vi "Get Next.vi"(0 "Subroutine in":refnum<class "Subroutine.lvclass">, 1 "Linked List Ref":refnum<data-value>, 5 "Active Unique ID":string, 9 "Active Element Index":i32, 11 "error in (no error)":errorcluster) -> (3 "Linked List Ref out":refnum<data-value>, 4 "Executioner out":refnum<class "Executioner.lvclass">, 6 "Active Unique ID out":string, 8 "Test Executive Ref out":refnum<data-value>, 10 "Active Element Index out":i32, 12 "Found":bool, 13 "Complete":bool, 14 "Stop":bool, 15 "error out":errorcluster)   [LabVIEW 2017, in "Custom Type Test Executive.lvlib" / "Subroutine.lvclass"]
uses:
  <vilib>/gpm_packages/@cs/test-executive/Source/Custom Type Test Executive/Subroutine/Subroutine.lvclass
  C:/Program Files/National Instruments/LabVIEW 2017/vi.lib/gpm_packages/@cs/test-executive/Source/Test Executive/Executioner/Executioner.lvclass
  <vilib>/gpm_packages/@cs/test-executive/Source/Test Executive/Executioner/Executioner.lvclass
  <vilib>/gpm_packages/@cs/linked-list/Source/Linked List/ILinkedList/ILinked List.lvclass
  <vilib>/gpm_packages/@cs/test-executive/Source/Test Executive/ITestExecutive/ITest Executive.lvclass
  <vilib>/gpm_packages/@cs/test-executive/Source/Custom Type Test Executive/Test Executive Data Type/Test Executive.lvclass/Test Executive.ctl
  <vilib>/gpm_packages/@cs/data-type-serializer/source/String/String.lvclass/String.ctl
  8685ad62-a5f1-424e-9210-060c18869b42.vi
  73af2345-b58a-4bc3-bab0-c6c44c39e3df.vi
  cb17b2c6-08af-4f3d-87c2-f0635200e88a.vi
  b989164a-f16b-4661-a128-dada9db9fdaa.vi
  56bd1768-b4b8-4ab7-8904-4290c8f45432.vi
  0b71244f-90f5-4307-84d1-8667a03d3b22.vi
  <vilib>/gpm_packages/@cs/test-executive/Source/Custom Type Test Executive/Test Executive Data Type/Test Executive.lvclass
  C:/Program Files/National Instruments/LabVIEW 2017/vi.lib/gpm_packages/@cs/data-type-serializer/source/Data Type/Data Type.lvclass
  <vilib>/gpm_packages/@cs/data-type-serializer/source/String/String.lvclass
  <vilib>/Utility/error.llb/Error Cluster From Error Code.vi
  <vilib>/gpm_packages/@cs/linked-list/Source/Linked List/Linked List Ref/Linked List Ref.lvclass
  <vilib>/gpm_packages/@cs/test-executive/Source/Test Executive/TestExecutive Ref/TestExecutive Ref.lvclass
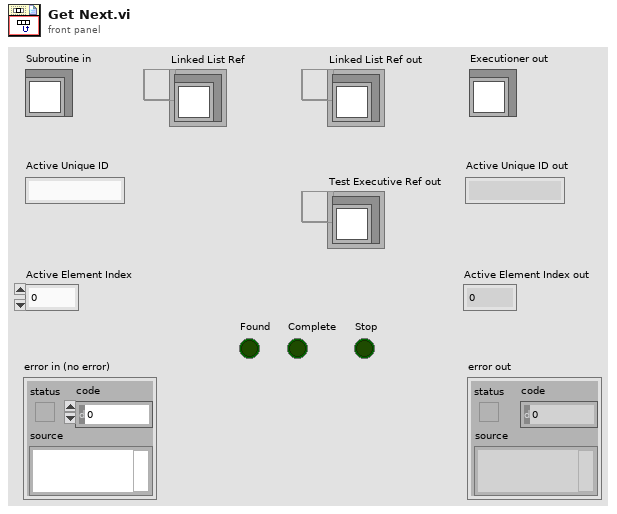
[diagram p1: front panel]
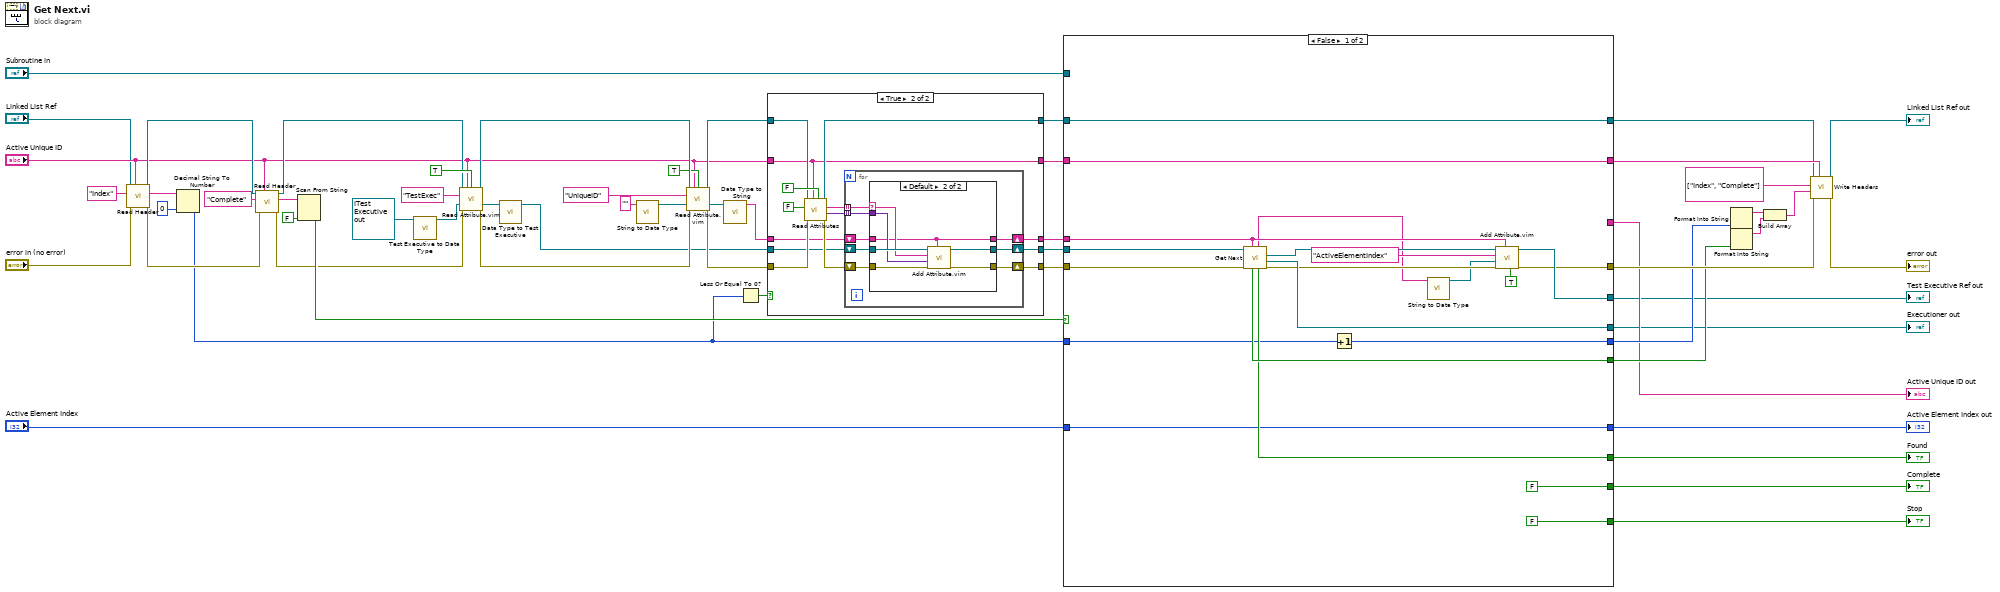
[diagram p0: block diagram]
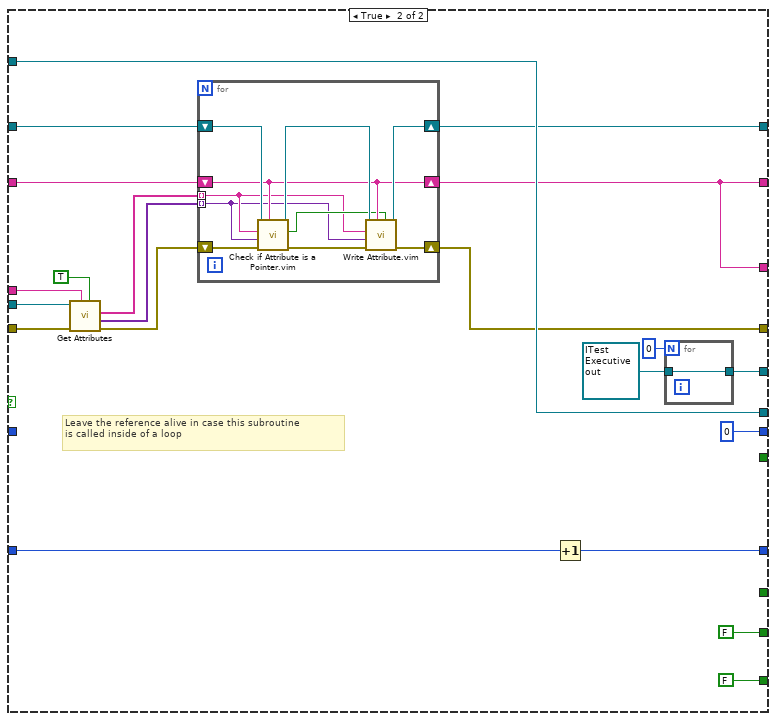
[diagram p4: hidden frame]
diagram:
  n1 = call <vilib>:"Read Header.vi"("Linked List ID"="Active Unique ID", "error in (no error)"="error in (no error)", "Header Name"="Index" ("Attribute Name"), "Linked List Ref"="Linked List Ref") -> ("error out"=w44:errorcluster, "Header Value"=w50:string, "Linked List Ref out"=w45:refnum<data-value>)  [unwired: 4 in, 1 out]
  n2 = Decimal String To Number(string=w50, default (0L)=0 ("Attribute")) -> (number=w23:i32)  [unwired: 1 in, 1 out]
  n3 = call <vilib>:"Read Header.vi"("Linked List ID"="Active Unique ID", "error in (no error)"=w44, "Header Name"="Complete" ("Attribute Name"), "Linked List Ref"=w45) -> ("error out"=w32:errorcluster, "Header Value"=w47:string, "Linked List Ref out"=w33:refnum<data-value>)  [unwired: 4 in, 1 out]
  n4 = Scan From String(input string=w47, default 1=FALSE) -> (output 1=w52:bool)  [unwired: 3 in, 3 out]
  n5 = call <vilib>:"Test Executive to Data Type.vi"("Test Executive Ref"=refnum<data-value> refnum ("Test Executive Ref out")) -> ("Boolean out"=w3:refnum<class "Test Executive.lvclass">)  [unwired: 9 in, 1 out]
  n6 = call "Read Attribute.vim"("Linked List Ref"=w33, "Linked List ID"="Active Unique ID", "Include Private?"=TRUE, "Attribute Name"="TestExec", "Type"=w3, "error in (no error)"=w32) -> ("Linked List Ref out"=w37:refnum<data-value>, "Attribute"=w2:refnum<class "Test Executive.lvclass">, "error out"=w35:errorcluster)  [unwired: 4 in, 3 out]
  n7 = call <vilib>:"Data Type to Test Executive.vi"("Data Type"=w2) -> ("Test Executive Ref"=w1:refnum<data-value>)  [unwired: 9 in, 1 out]
  n8 = call <vilib>:"String to Data Type.vi"("String"="") -> ("Boolean out"=w7:refnum<class "String.lvclass">)  [unwired: 9 in, 1 out]
  n9 = call "Read Attribute.vim"("Linked List Ref"=w37, "Linked List ID"="Active Unique ID", "Include Private?"=TRUE, "Attribute Name"="UniqueID", "Type"=w7, "error in (no error)"=w35) -> ("Linked List Ref out"=w27:refnum<data-value>, "Attribute"=w6:refnum<class "String.lvclass">, "error out"=w31:errorcluster)  [unwired: 4 in, 3 out]
  n10 = call <vilib>:"Data Type to String.vi"("Data Type"=w6) -> ("String out"=w5:string)  [unwired: 9 in, 1 out]
  n11 = Less Or Equal To 0?(x=w23) -> (x <= 0?=w24:bool)
  n12 = case shown="True" w24 {
    tunnel: "Active Unique ID" -> [w58 w63]
    tunnel: w31 -> [w60 w71]
    tunnel: [w60 w70] -> w30
    tunnel: w5 -> [w59 w69]
    tunnel: [w59 w68] -> w29
    tunnel: w1 -> [w61 w67]
    tunnel: [w61 w66] -> w28
    tunnel: w27 -> [w62 w65]
    tunnel: [w62 w64] -> w26
    tunnel: [w58 w63] -> w25
    frame False {
    }
    frame True {
      n13 = call <vilib>:"Read Attributes.vi"("Flatten Pointer?"=FALSE, "Linked List ID"=w63, "error in (no error)"=w71, "Include Private?"=FALSE, "Linked List Ref"=w65) -> ("error out"=w75:errorcluster, "Attributes"=w72:variant[], "Attribute Names out"=w74:string[], "Linked List Ref out"=w64:refnum<data-value>)  [unwired: 1 in, 2 out]
      n14 = for {
        shift-right: [w81] -> w70
        shift-left: w75 -> [w82]
        tunnel: w74 -> [w80] mode=indexing
        tunnel: w72 -> [w79] mode=indexing
        shift-right: [w78] -> w68
        shift-left: w69 -> [w83]
        shift-right: [w77] -> w66
        shift-left: w67 -> [w84]
        n15 = case shown="Default" w80 {
          selector: w80 -> [_ w91]
          tunnel: w84 -> [w85 w94]
          tunnel: w83 -> [w86 w89]
          tunnel: w82 -> [w87 w93]
          tunnel: [w87 w92] -> w81
          tunnel: w79 -> [_ w90]
          tunnel: [w86 w89] -> w78
          tunnel: [w85 w88] -> w77
          frame "Restore Point" {
          }
          frame Default {
            n16 = call "Add Attribute.vim"("ID"=w89, "error in (no error)"=w93, "Attribute"=w90, "Attribute Name"=w91, "Test Executive Ref"=w94) -> ("error out"=w92:errorcluster, "Test Executive Ref out"=w88:refnum<data-value>)  [unwired: 3 in, 2 out]
          }
        }
      }
    }
  }
  n17 = case shown="False" w52 {
    tunnel: w28 -> [w115 w127]
    tunnel: [w108 w135] -> w12
    tunnel: [w114 _] -> w53
    tunnel: [w105 w121] -> w13
    tunnel: [w113 w123] -> w56
    tunnel: w26 -> [w113 w124]
    tunnel: [w97 0] -> w54
    tunnel: w23 -> [w109 _]
    tunnel: [w112 _] -> w15
    tunnel: [FALSE FALSE] -> w16
    tunnel: [w111 w133] -> w14
    tunnel: "Active Element Index" -> [w111 w136]
    tunnel: "Subroutine in" -> [_ w135]
    tunnel: w30 -> [w110 w126]
    tunnel: [w105 w121] -> w57
    tunnel: w25 -> [w105 w122]
    tunnel: [w101 w116] -> w55
    tunnel: w29 -> [w100 w125]
    tunnel: [w103 w130] -> w10
    tunnel: [FALSE FALSE] -> w17
    frame False {
      n18 = call <vilib>:"Get Next.vi"("Unique ID"=w100, "error in (no error)"=w110, "Test Executive Ref"=w115) -> ("error out"=w102:errorcluster, "Test"=w108:refnum<class "Executioner.lvclass">, "Active Test Executive Ref out"=w104:refnum<data-value>, "Found"=w112:bool, "Unique ID out"=w96:string, "Complete"=w114:bool)  [unwired: 2 in, 1 out]
      n19 = Increment(x=w109) -> (x+1=w97:i32)
      n20 = call <vilib>:"String to Data Type.vi"("String"=w96) -> ("Boolean out"=w95:refnum<class "String.lvclass">)  [unwired: 9 in, 1 out]
      n21 = call "Add Attribute.vim"("Private?"=TRUE, "ID"=w100, "error in (no error)"=w102, "Attribute"=w95, "Attribute Name"="ActiveElementIndex", "Test Executive Ref"=w104) -> ("error out"=w101:errorcluster, "Test Executive Ref out"=w103:refnum<data-value>)  [unwired: 2 in, 2 out]
    }
    frame True {
      # "Leave the reference alive in case this subroutine\nis called inside of a loop"
      n22 = call <vilib>:"Get Attributes.vi"("Flatten Pointer?"=TRUE, "Test ID"=w125, "error in (no error)"=w126, "Test Executive Ref"=w127) -> ("error out"=w118:errorcluster, "Attributes"=w119:variant[], "Attribute Names out"=w120:string[])  [unwired: 2 in, 3 out]
      n23 = for {
        shift-right: [w141] -> w123
        shift-left: w124 -> [w146]
        shift-right: [w140] -> w121
        shift-left: w122 -> [w140]
        tunnel: w120 -> [w138] mode=indexing
        tunnel: w119 -> [w137] mode=indexing
        shift-right: [w143] -> w116
        shift-left: w118 -> [w145]
        n24 = call "Check if Attribute is a Pointer.vim"("Linked List ID"=w140, "error in (no error)"=w145, "Type"=w137, "Attribute Name"=w138, "Linked List Ref"=w146) -> ("error out"=w144:errorcluster, "Pointer?"=w139:bool, "Linked List Ref out"=w142:refnum<data-value>)  [unwired: 2 in, 2 out]
        n25 = call "Write Attribute.vim"("Update Pointer?"=w139, "Linked List ID"=w140, "error in (no error)"=w144, "Attribute"=w137, "Attribute Name"=w138, "Linked List Ref"=w142) -> ("error out"=w143:errorcluster, "Linked List Ref out"=w141:refnum<data-value>)  [unwired: 2 in, 2 out]
      }
      n26 = Increment(x=w136) -> (x+1=w133:i32)
      n27 = for {
        N: 0 -> [_]
        tunnel: refnum<data-value> refnum ("Test Executive Ref out") -> [w147]
        tunnel: [w147] -> w130
      }
    }
  }
  "Executioner out" <- w12
  "Active Unique ID out" <- w13
  "Active Element Index out" <- w14
  "Found" <- w15
  "Complete" <- w16
  "Stop" <- w17
  "Test Executive Ref out" <- w10
  n28 = Format Into String(w54) -> (resulting string=w42:string)  [unwired: 3 in, 1 out]
  n29 = Format Into String(w53) -> (resulting string=w40:string)  [unwired: 3 in, 1 out]
  n30 = Build Array(w42, w40) -> (w41:string[])
  n31 = call <vilib>:"Write Headers.vi"("Linked List ID"=w57, "error in (no error)"=w55, "Header Values"=w41, "Header Names"=string[] ["Index", "Complete"], "Linked List Ref"=w56) -> ("error out"=→"error out":errorcluster, "Linked List Ref out"=→"Linked List Ref out":refnum<data-value>)  [unwired: 5 in]
